vi "Mirror Image(8 bit Vertical).vi"(8 "错误输入":errorcluster, 11 "image In":T1 caption="Image in") -> (0 "错误输出":errorcluster, 3 "image out":T1 caption="Image out")   [LabVIEW 2012, in "Picture Box Tools.lvlib"]
uses:
  <vilib>/picture/picture.llb/imagedata.ctl
  Picture Box Tools.lvlib
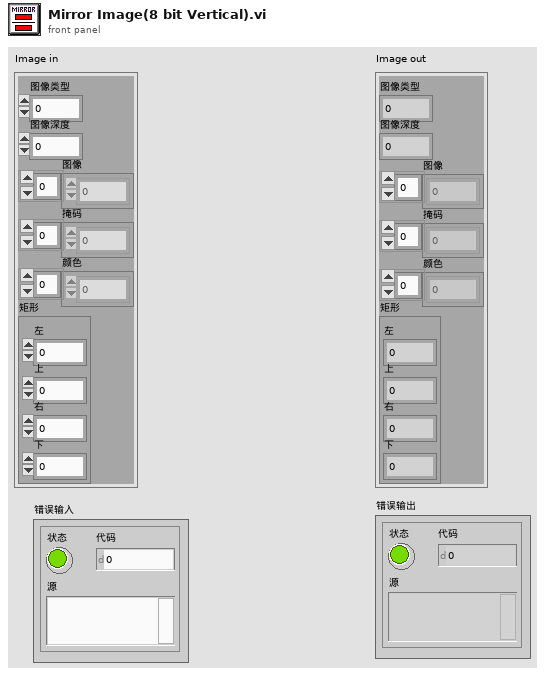
[diagram p1: front panel]
types:
  T1 = typedef "imagedata.ctl" = cluster{"image type":i32, "image depth":i32, "image":u8[], "mask":u8[], "colors":u32[], "Rectangle":cluster{"left":i16, "top":i16, "right":i16, "bottom":i16}}
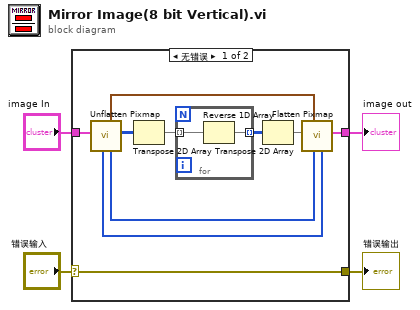
[diagram p0: block diagram]
diagram:
  n1 = case shown="无错误" "错误输入" {
    selector: "错误输入" -> [w11 w17]
    tunnel: [w11 w17] -> w3
    tunnel: "image In" -> [w10 _]
    tunnel: [w9 _] -> w1
    frame No Error {
      n2 = call <vilib>:"Unflatten Pixmap.vi"("image data"=w10) -> ("8-bit pixmap"=w6:u8[][], "colors"=w14:u32[], "top left"=w12:cluster{"x":i16, "y":i16}, "mask"=w13:u8[])  [unwired: 4 in, 3 out]
      n3 = Transpose 2D Array(2D array=w6) -> (transposed array=w7:u8[][])
      n4 = for {
        tunnel: w7 -> [w16] mode=indexing
        tunnel: [w15] -> w8 mode=indexing
        n5 = Reverse 1D Array(array=w16) -> (reversed array=w15:u8[])
      }
      n6 = Transpose 2D Array(2D array=w8) -> (transposed array=w5:u8[][])
      n7 = call <vilib>:"Flatten Pixmap.vi"("mask"=w13, "colors"=w14, "top left"=w12, "8-bit pixmap"=w5) -> ("image data"=w9:T1)  [unwired: 7 in]
    }
    frame Error {
    }
  }
  "错误输出" <- w3
  "image out" <- w1
